vi "Computer Main.vi"() -> ()   [LabVIEW 2011]
doc: "This VI imlements the framework and scheduler for your robotics program. It should not be necessary to modify the framework. You are expected to add your code to the VIs called from Robot Main, the ones located in the Team Code within the project."
panel:
  out "Found Target":bool
  out "Bounding Rect":T1
  out "Ready":bool
  out "Elevation Angle":dbl=30.25583
  out "Shortest Dist To Rect Center":dbl=-76.74527606681221
  out "Offset Angle From Perpendicular":dbl=-20.25
  in  "Take Pics":bool
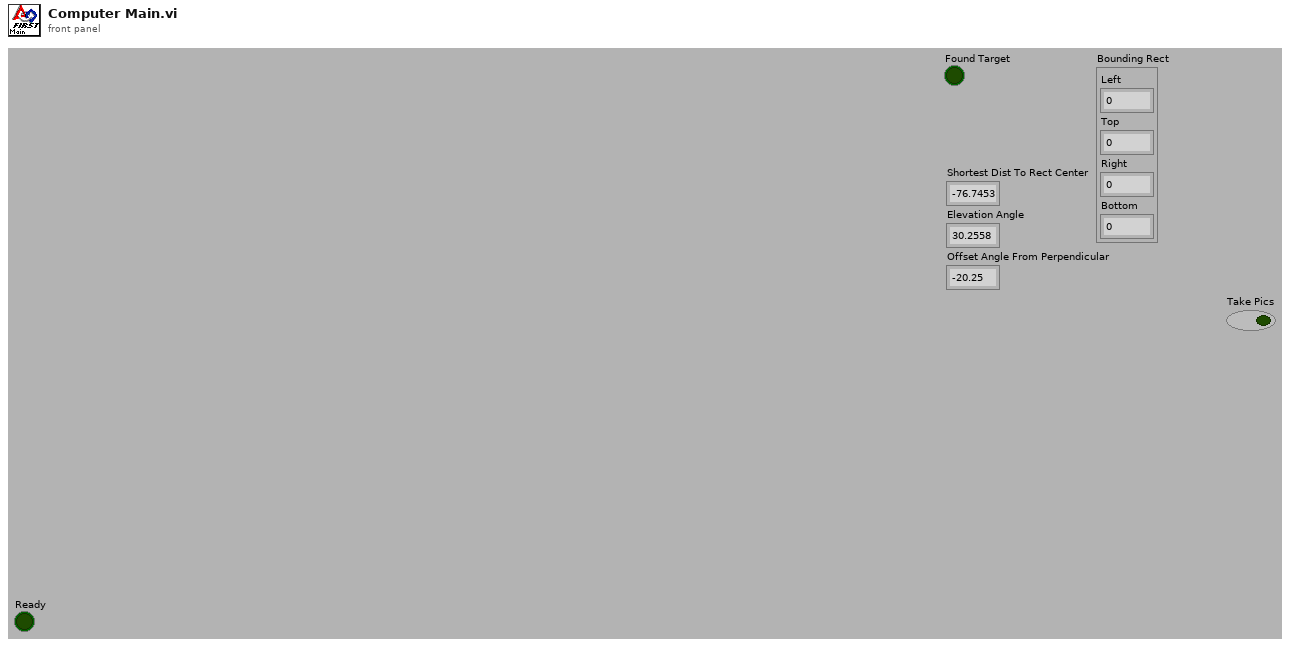
[diagram p1: front panel]
types:
  T1 = cluster{"Left":dbl, "Top":dbl, "Right":dbl, "Bottom":dbl}
  T2 = typedef "WPI_CameraDevRef.ctl" = cluster{"Camera Address":string, "CameraStatus":errorcluster, "Acquire Image Notifier":refnum<notifier>}
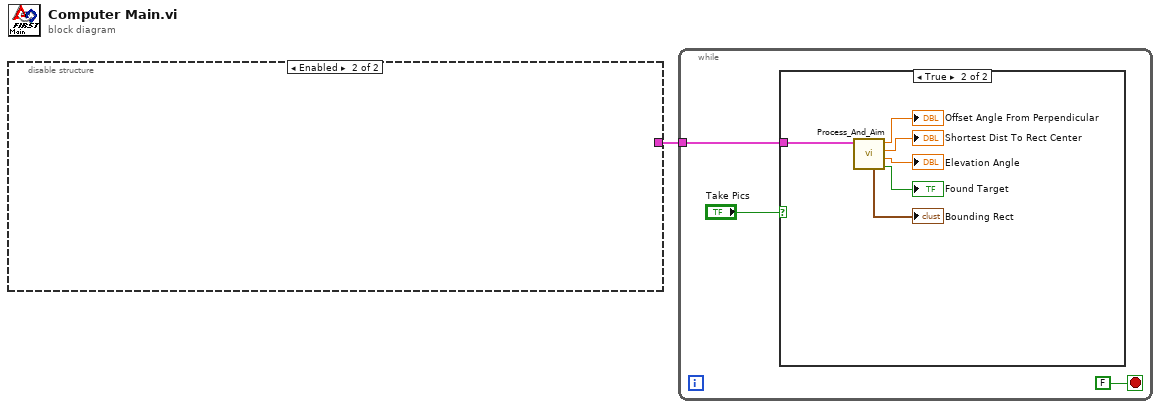
[diagram p0: block diagram]
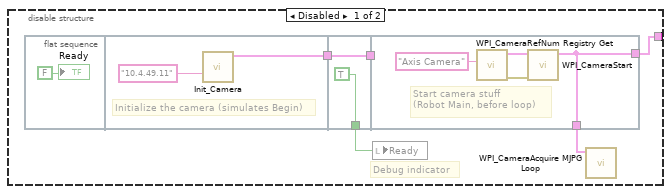
[diagram p2: hidden frame]
diagram:
  n1 = disable-structure shown="Enabled" {
    disable-tunnel: [w3 _] -> w1
    frame Disabled {
      # "Debug indicator"
      n2 = flat-sequence {
        tunnel: [w8] -> w6
        tunnel: w6 -> [w11]
        tunnel: [TRUE] -> w5
        tunnel: [w11] -> w4
        tunnel: w4 -> [_]
        tunnel: [w12] -> w3
        tunnel: [w12] -> w2
        frame #0 {
          "Ready" <- FALSE
        }
        frame #1 {
          # "Initialize the camera (simulates Begin)"
          n3 = call "Init_Camera.vi"("Camera IP"="10.4.49.11") -> ("CameraDevRef Out"=w8:T2)  [unwired: 10 in]
        }
        frame #2 {
        }
        frame #3 {
          # "Start camera stuff\n(Robot Main, before loop)"
          n4 = call <vilib>:"WPI_CameraRefNum Registry Get.vi"("refnum name"="Axis Camera") -> ("error out"=w14:errorcluster, "CameraDevRef"=w15:T2)  [unwired: 9 in]
          n5 = call <vilib>:"WPI_CameraStart.vi"("error in (no error)"=w14, "CameraDevRef"=w15) -> ("CameraDevRef Out"=w12:T2)  [unwired: 8 in, 1 out]
        }
      }
      n6 = local write "Ready"(w5) -> ()
      n7 = call <vilib>:"WPI_CameraAcquire MJPG Loop.vi"("CameraDevRef"=w2) -> ()  [unwired: 11 in]
    }
    frame Enabled {
    }
  }
  n8 = while {
    tunnel: w1 -> [w18]
    stop <- FALSE stop-if-true
    n9 = case shown="True" "Take Pics" {
      tunnel: w18 -> [_ w24]
      frame False {
      }
      frame True {
        n10 = call "Process_And_Aim.vi"("CameraDevRef"=w24) -> ("Found Target"=→"Found Target":bool, "Elevation Angle"=→"Elevation Angle":dbl, "Target Dist"=→"Shortest Dist To Rect Center":dbl, "Offset Angle From Perpendicular"=→"Offset Angle From Perpendicular":dbl, "Bounding Rect"=→"Bounding Rect":T1)  [unwired: 6 in]
      }
    }
  }
